vi "WPI_Power Get roboRIO Rail Faults.vi"(11 "error in":errorcluster) -> (4 "Input Voltage Brown Out":bool, 6 "3.3V User Rail Short":bool, 8 "5 V User Rail Short":bool, 10 "6 V User Rail Short":bool, 14 "5V User Rail Brown Out":bool, 15 "error out":errorcluster)   [LabVIEW 2017]
doc: "Returns any rail faults on the roboRIO."
uses:
  <vilib>/Rock Robotics/SystemInterfaces/Power/FPGA_PowerStatus.ctl
  <vilib>/Utility/error.llb/Error Cluster From Error Code.vi
  <vilib>/rvi/errors/niLvFpgaAdjustHostInterfaceError.vi
  <vilib>/rvi/interface/nirviReadWriteControl/nirviReadWriteControl.xnode
  <vilib>/Rock Robotics/SystemInterfaces/System/FPGA_SystemFRC FPGA Ref.ctl
  NiFpgaLv.dll
  <vilib>/rvi/interface/Simulation/niFpgaSimulationCallBeginRW.vi
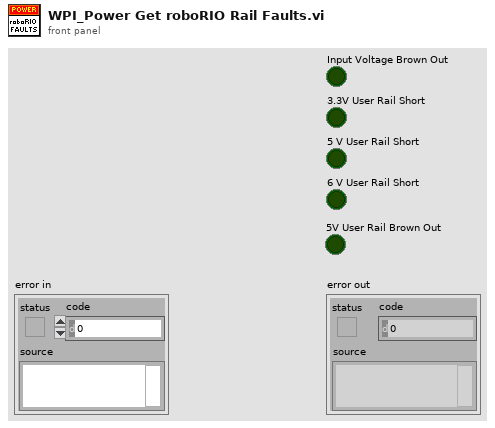
[diagram p1: front panel]
types:
  T1 = typedef "FPGA_PowerStatus.ctl" = enum8{"Disable", "Brownout", "Fault (Overcurrent)", "Fault (Voltage Out of Range)", "Power Good"}
  T2 = typedef "FPGA_SystemFRC FPGA Ref.ctl" = refnum<k20>
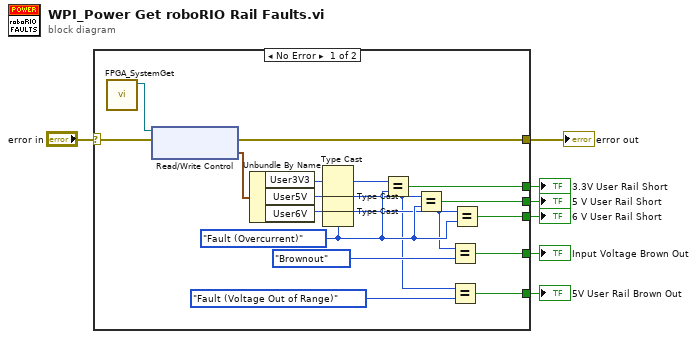
[diagram p0: block diagram]
diagram:
  n1 = case shown="No Error" "error in" {
    selector: "error in" -> [w24 w26]
    tunnel: [w23 w26] -> w6
    tunnel: [w16 _] -> w5
    tunnel: [w15 _] -> w4
    tunnel: [w14 _] -> w3
    tunnel: [w11 _] -> w2
    tunnel: [w8 _] -> w1
    frame No Error {
      w17 = FPGA_PowerStatus."Fault (Overcurrent)" ("Power Status")
      n2 = call <vilib>:"FPGA_SystemGet.vi"() -> ("FRC FPGA Ref"=w25:T2)  [unwired: 2 in, 9 out]
      n3 = xnode "Read/Write Control"("FPGA VI Reference In"=w25, "error in"=w24) -> ("error out"=w23:errorcluster, "Power.Status"=w22:cluster{"User3V3":u8, "User5V":u8, "User6V":u8})  [unwired: 1 out]
      n4 = Unbundle By Name(w22) -> ("User3V3"=w21:u8, "User5V"=w20:u8, "User6V"=w19:u8)
      n5 = Type Cast(type=w17, x=w21) -> (*(type *) &x=w18:T1)
      n6 = Type Cast(type=w17, x=w20) -> (*(type *) &x=w9:T1)
      n7 = Type Cast(type=w17, x=w19) -> (*(type *) &x=w13:T1)
      n8 = Equal?(x=w18, y=w17) -> (x = y?=w16:bool)
      n9 = Equal?(x=w9, y=w17) -> (x = y?=w15:bool)
      n10 = Equal?(x=w13, y=FPGA_PowerStatus."Brownout" ("Power Status")) -> (x = y?=w11:bool)
      n11 = Equal?(x=w9, y=FPGA_PowerStatus."Fault (Voltage Out of Range)" ("Power Status")) -> (x = y?=w8:bool)
      n12 = Equal?(x=w13, y=w17) -> (x = y?=w14:bool)
    }
    frame Error {
    }
  }
  "error out" <- w6
  "3.3V User Rail Short" <- w5
  "5 V User Rail Short" <- w4
  "6 V User Rail Short" <- w3
  "Input Voltage Brown Out" <- w2
  "5V User Rail Brown Out" <- w1
